vi "Write Trig Params.vi"(8 "error in":errorcluster, 9 "Ctrl Interval":dbl, 10 "Trig Resolution":u32, 11 "Config and Run TRIG Process in":refnum<class "Config and Run TRIG Process.lvclass">) -> (0 "error out":errorcluster, 3 "Config and Run TRIG Process out":refnum<class "Config and Run TRIG Process.lvclass">)   [LabVIEW 2019, in "Trig Process.lvlib" / "Config and Run TRIG Process.lvclass"]
uses:
  Config and Run TRIG Process.lvclass
  Config and Run TRIG Process.lvclass/Config and Run TRIG Process.ctl
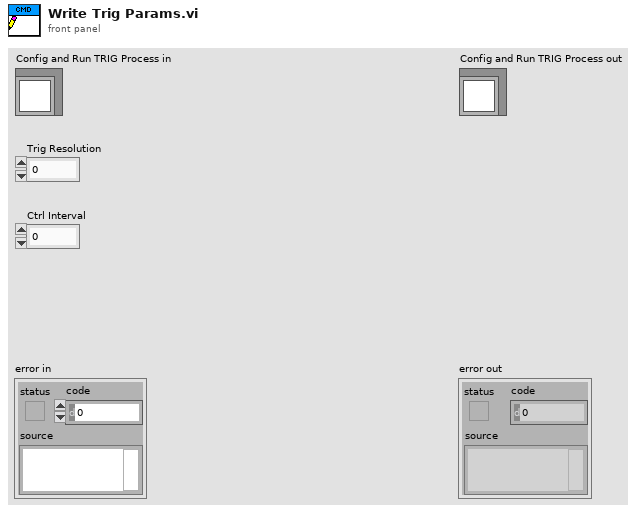
[diagram p1: front panel]
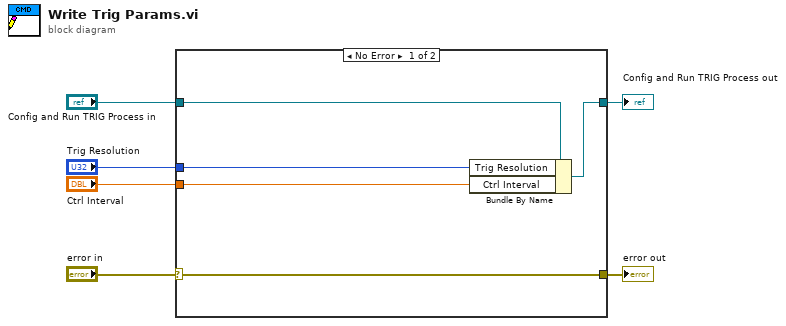
[diagram p0: block diagram]
diagram:
  n1 = case shown="No Error" "error in" {
    selector: "error in" -> [w11 w12]
    tunnel: [w11 w12] -> w5
    tunnel: [w9 w13] -> w3
    tunnel: "Config and Run TRIG Process in" -> [w10 w13]
    tunnel: "Trig Resolution" -> [w8 _]
    tunnel: "Ctrl Interval" -> [w7 _]
    frame No Error {
      n2 = Bundle By Name(cluster=w10, "Trig Resolution"=w8, "Ctrl Interval"=w7) -> (w9:refnum<class "Config and Run TRIG Process.lvclass">)
    }
    frame Error {
    }
  }
  "error out" <- w5
  "Config and Run TRIG Process out" <- w3
